vi "GetWaveformRegistrations.vi"(8 "error in (no error)":errorcluster, 10 "acquisition channels (in acquisition order)":T12[](array[typedef]), 11 "device":T4) -> (0 "error out":errorcluster, 1 "register data sets":T1[](array[typedef]))   [LabVIEW 2017, in "McsaFpgaAcquisition.lvlib"]
uses:
  <vilib>/addons/InsightCM/Devices/Shared/Mcsa/McsaFpgaAcquisition/McsaFpgaAcquisition.lvlib
  <vilib>/addons/InsightCM/MessageBus/Base/controls/R2_Channel.ctl
  <vilib>/addons/InsightCM/MessageBus/Base/controls/KeyValuePair.ctl
  <vilib>/addons/InsightCM/MessageBus/Base/controls/Metric.ctl
  <vilib>/addons/InsightCM/MessageBus/Base/controls/R2_Device.ctl
  <vilib>/addons/InsightCM/MessageBus/Base/controls/DeviceState.ctl
  <vilib>/addons/InsightCM/MessageBus/Base/controls/R2_DataGroup.ctl
  <vilib>/addons/InsightCM/MessageBus/Base/controls/OperatingState.ctl
  <vilib>/addons/InsightCM/MessageBus/Base/controls/Trigger.ctl
  <vilib>/addons/InsightCM/MessageBus/Base/controls/Condition.ctl
  <vilib>/addons/InsightCM/MessageBus/Base/controls/BurstModeTrigger.ctl
  <vilib>/addons/InsightCM/Devices/Shared/Mcsa/McsaDataEventCreator/controls/RegisterDataSets.ctl
  <vilib>/addons/InsightCM/Devices/Shared/Mcsa/McsaDataEventCreator/controls/Registry_DataSet.ctl
  <vilib>/addons/InsightCM/Devices/Shared/Mcsa/McsaDataEventCreator/controls/DataSetType.ctl
  <vilib>/addons/InsightCM/MessageBus/Base/controls/R2_DeviceModel.ctl
  <vilib>/addons/InsightCM/MessageBus/Base/controls/Tag.ctl
  <vilib>/addons/InsightCM/Utilities/DeviceModelHelpers/DeviceModelHelpers.lvlib
  <vilib>/addons/InsightCM/Devices/Shared/Mcsa/McsaDataEventCreator/McsaDataEventCreator.lvlib
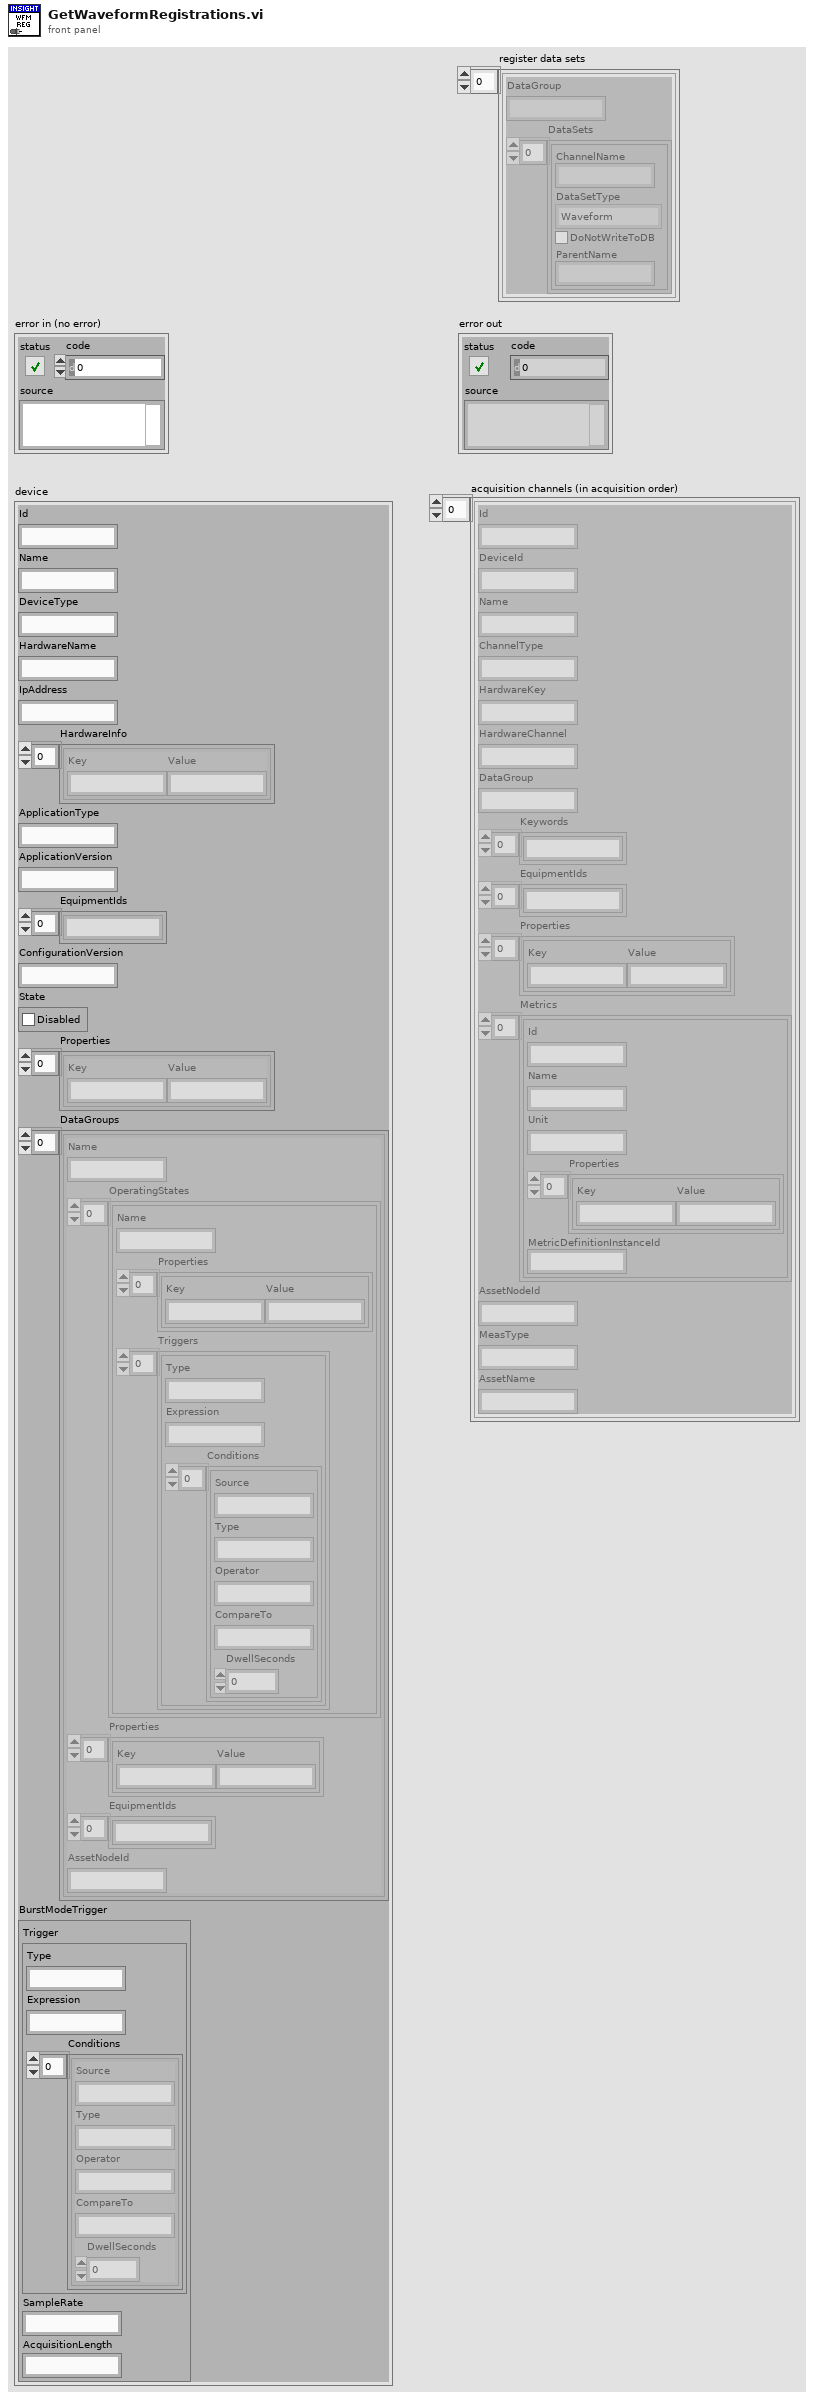
[diagram p1: front panel]
types:
  T1 = typedef "McsaDataEventCreator.lvlib/RegisterDataSets.ctl" = cluster{"DataGroup":string, "DataSets":T2[]}
  T2 = typedef "McsaDataEventCreator.lvlib/Registry_DataSet.ctl" = cluster{"ChannelName":string, "DataSetType":T3, "DoNotWriteToDB":bool, "ParentName":string}
  T3 = typedef "McsaDataEventCreator.lvlib/DataSetType.ctl" = enum16{"Waveform", "MCSAFFT", "TorqueWFM"}
  T4 = typedef "R2_Device.ctl" = cluster{"Id":string, "Name":string, "DeviceType":string, "HardwareName":string, "IpAddress":string, "HardwareInfo":T5[], "ApplicationType":string, "ApplicationVersion":string, "EquipmentIds":string[], "ConfigurationVersion":string, "State":T6, "Properties":T5[], "DataGroups":T7[], "BurstModeTrigger":T11}
  T5 = typedef "KeyValuePair.ctl" = cluster{"Key":string, "Value":string}
  T6 = typedef "DeviceState.ctl" = cluster{"Disabled":bool}
  T7 = typedef "R2_DataGroup.ctl" = cluster{"Name":string, "OperatingStates":T8[], "Properties":T5[], "EquipmentIds":string[], "AssetNodeId":string}
  T8 = typedef "OperatingState.ctl" = cluster{"Name":string, "Properties":T5[], "Triggers":T9[]}
  T9 = typedef "Trigger.ctl" = cluster{"Type":string, "Expression":string, "Conditions":T10[]}
  T10 = typedef "Condition.ctl" = cluster{"Source":string, "Type":string, "Operator":string, "CompareTo":string, "DwellSeconds":dbl}
  T11 = typedef "BurstModeTrigger.ctl" = cluster{"Trigger":T9, "SampleRate":string, "AcquisitionLength":string}
  T12 = typedef "R2_Channel.ctl" = cluster{"Id":string, "DeviceId":string, "Name":string, "ChannelType":string, "HardwareKey":string, "HardwareChannel":string, "DataGroup":string, "Keywords":string[], "EquipmentIds":string[], "Properties":T5[], "Metrics":T13[], "AssetNodeId":string, "MeasType":string, "AssetName":string}
  T13 = typedef "Metric.ctl" = cluster{"Id":string, "Name":string, "Unit":string, "Properties":T5[], "MetricDefinitionInstanceId":string}
  T14 = typedef "R2_DeviceModel.ctl" = cluster{"Device":T4, "Channels":T12[], "Tags":T15[]}
  T15 = typedef "Tag.ctl" = cluster{"Id":string, "Path":string, "Name":string, "Datatype":string, "Props":T5[], "Keywords":string[]}
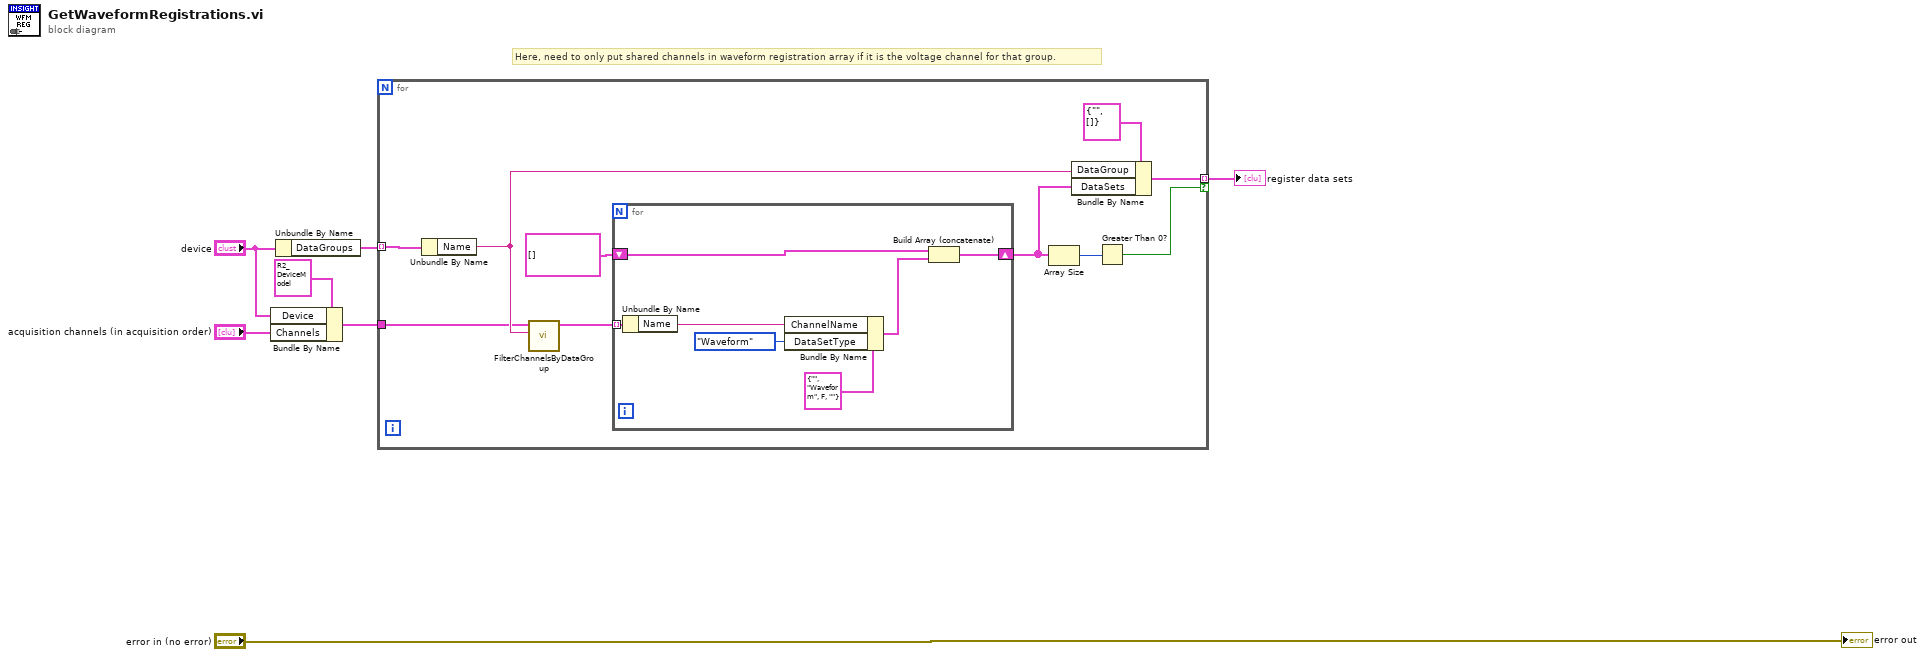
[diagram p0: block diagram]
diagram:
  # "Here, need to only put shared channels in waveform registration array if it is the voltage channel for that group."
  n1 = Bundle By Name(cluster=T14 {"Device"={"Id"="", "Name"="", "DeviceType"="", "HardwareName"="", "IpAddress"="", "HardwareInfo"=[], "ApplicationType"="", "ApplicationVersion"="", "EquipmentIds"=[], "ConfigurationVersion"="", "State"={"Disabled"=FALSE}, "Properties"=[], "DataGroups"=[], "BurstModeTrigger"={"Trigger"={"Type"="", "Expression"="", "Conditions"=[]}, "SampleRate"="", "AcquisitionLength"=""}}, "Channels"=[], "Tags"=[]} ("device model"), "Device"="device", "Channels"="acquisition channels (in acquisition order)") -> (w2:T14)
  n2 = Unbundle By Name("device") -> ("DataGroups"=w7:T7[])
  n3 = for {
    tunnel: w7 -> [w12] mode=indexing
    tunnel: [w17] -> w1 mode=indexing if=w15
    tunnel: w2 -> [w13]
    n4 = Unbundle By Name(w12) -> ("Name"=w14:string)
    n5 = call <vilib>:"FilterChannelsByDataGroup.vi"("group"=w14, "device model"=w13) -> ("channels in data group"=w11:T12[])  [unwired: 8 in, 1 out]
    n6 = for {
      tunnel: w11 -> [w24] mode=indexing
      shift-right: [w21] -> w8
      shift-left: T2[] [] -> [w22]
      n7 = Unbundle By Name(w24) -> ("Name"=w23:string)
      n8 = Bundle By Name(cluster=T2 {"ChannelName"="", "DataSetType"=enum."Waveform", "DoNotWriteToDB"=FALSE, "ParentName"=""} ("DataSet"), "ChannelName"=w23, "DataSetType"=DataSetType."Waveform") -> (w18:T2)
      n9 = Build Array (concatenate)(w22, w18) -> (w21:T2[])
    }
    n10 = Array Size(array=w8) -> (size(s)=w16:i32)
    n11 = Bundle By Name(cluster=T1 {"DataGroup"="", "DataSets"=[]} ("RegisterDataSet"), "DataGroup"=w14, "DataSets"=w8) -> (w17:T1)
    n12 = Greater Than 0?(x=w16) -> (x > 0?=w15:bool)
  }
  "register data sets" <- w1
  "error out" <- "error in (no error)"
